vi "MSScript_Act_BlockComment.vi"(8 "error in (no error)":errorcluster, 11 "MSScript in":refnum<class "MSScript.lvclass">) -> (0 "error out":errorcluster, 3 "MSScript out":refnum<class "MSScript.lvclass">)   [LabVIEW 2018, in "MSScript.lvclass"]
uses:
  MSScript.lvclass
  MSScript.lvclass/MSScript.ctl
  MSScript_Error_(6010)CommentLost.vi
  <vilib>/regexp/Match Regular Expression.xnode
panel:
  out "Array":string[](array[string])
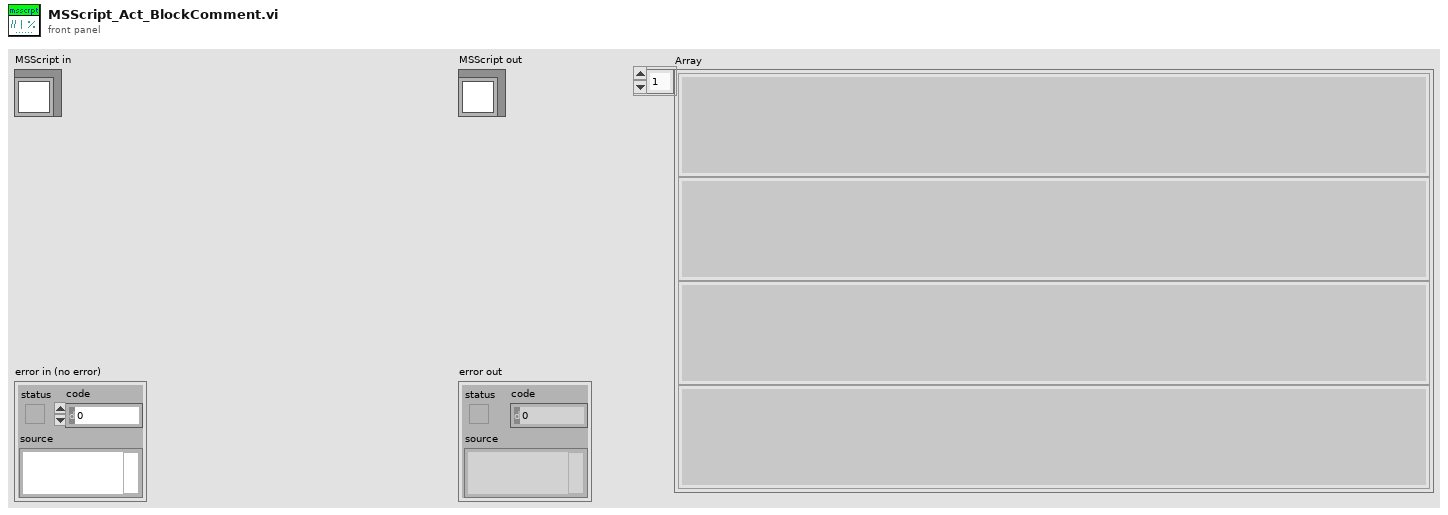
[diagram p1: front panel]
types:
  T1 = cluster{"Colour":u32, "Italic":bool, "Bold":bool}
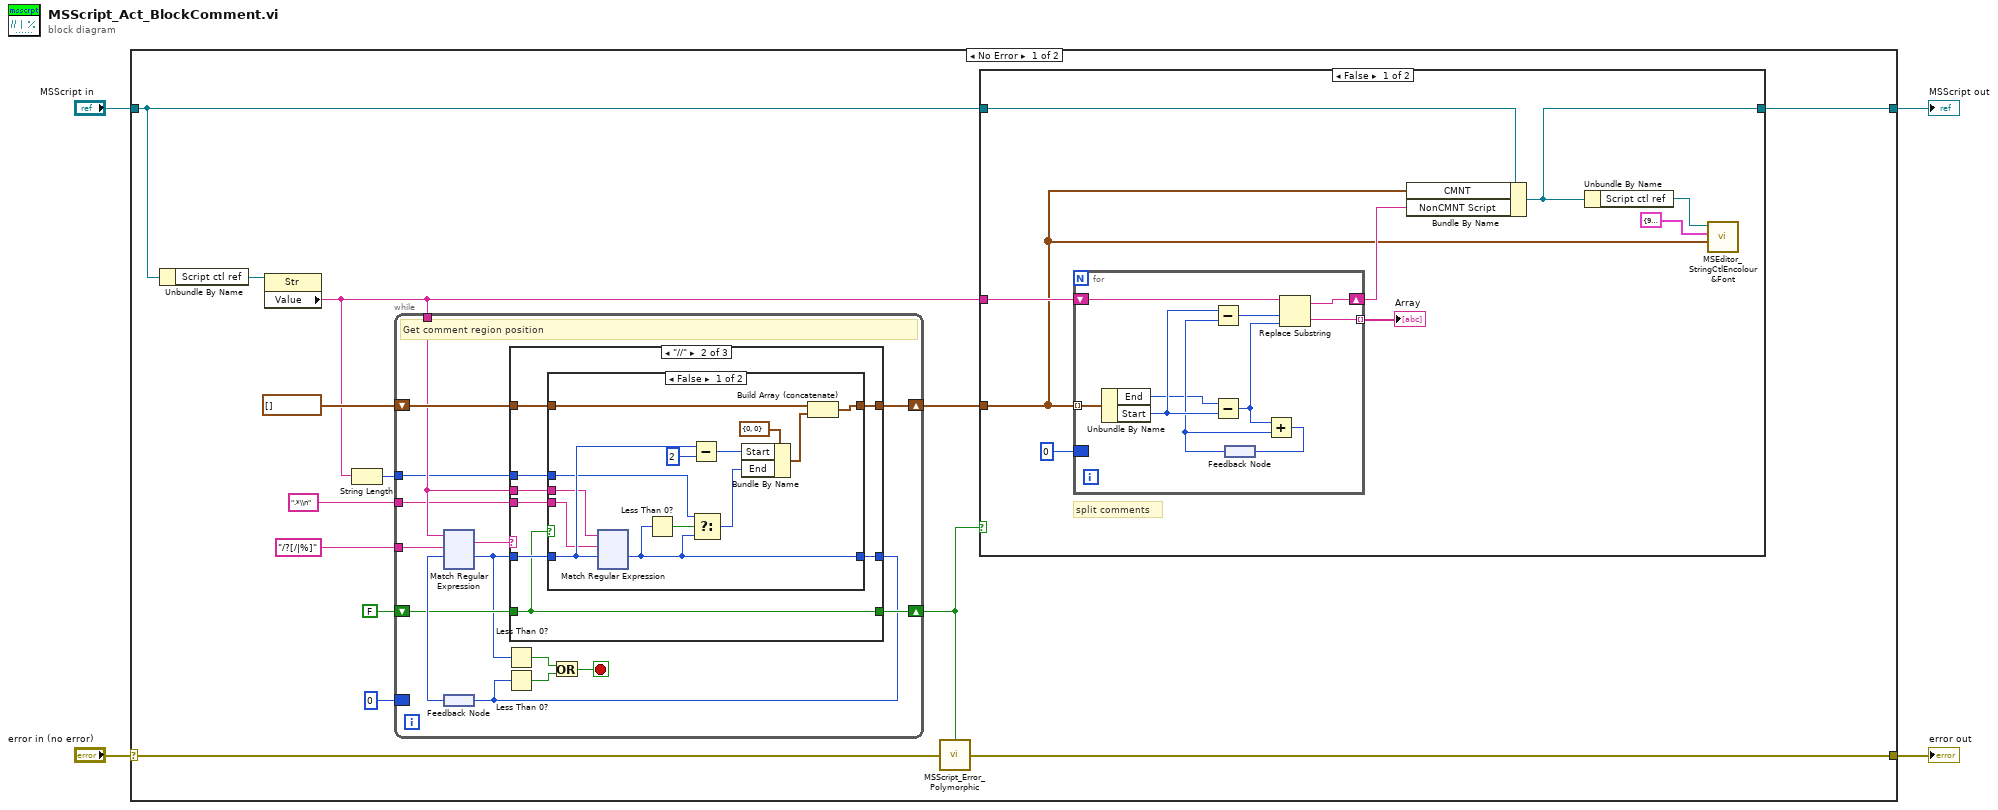
[diagram p0: block diagram]
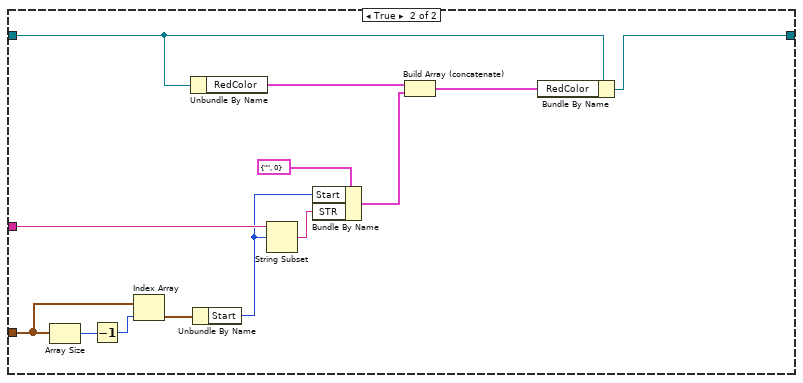
[diagram p2: hidden frame]
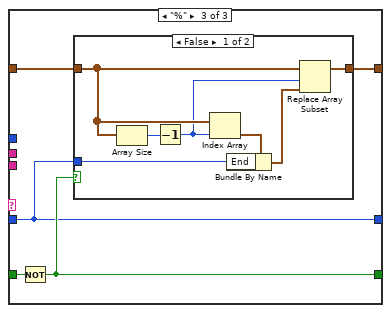
[diagram p5: hidden frame]
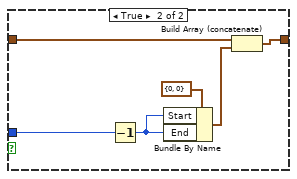
[diagram p6: hidden frame]
diagram:
  n1 = case shown="No Error" "error in (no error)" {
    selector: "error in (no error)" -> [w9 w339]
    tunnel: [w8 w339] -> w3
    tunnel: [w7 w338] -> w1
    tunnel: "MSScript in" -> [w6 w338]
    frame No Error {
      n2 = Unbundle By Name(w6) -> ("Script ctl ref"=w18:refnum<vi>)
      n3 = property class="Str"(reference=w18) -> ("Value"=w11:string)  [unwired: 1 in, 2 out]
      n4 = String Length(string=w11) -> (length=w12:i32)
      n5 = while {
        border: 0 ("offset past match") -> [_]
        tunnel: "/?[/|%]" ("regular expression") -> [w64]
        shift-right: [w61] -> w5
        shift-left: FALSE -> [w62]
        shift-right: [w58] -> w10
        shift-left: cluster{"Start":i32, "End":i32}[] [] ("Comments") -> [w60]
        tunnel: w11 -> [w57]
        tunnel: ".*\\n" ("regular expression") -> [w56]
        tunnel: w12 -> [w55]
        stop <- w51 stop-if-true
        # "Get comment region position"
        n6 = feedback #1() -> (w65:i32)
        n7 = xnode "Match Regular Expression"("input string"=w57, "regular expression"=w64, "offset (0)"=w65) -> ("whole match"=w63:string, "offset past match"=w59:i32)  [unwired: 3 in, 3 out]
        n8 = Less Than 0?(x=w59) -> (x < 0?=w53:bool)
        n9 = case shown="\"//\"" w63 {
          tunnel: w62 -> [w67 w71 w210]
          tunnel: [w67 w71 w209] -> w61
          tunnel: w60 -> [w66 w75 w207]
          tunnel: w57 -> [_ w76 _]
          tunnel: w59 -> [w68 w73 w208]
          tunnel: [w68 w72 w208] -> w54
          tunnel: [w66 w74 w206] -> w58
          tunnel: w56 -> [_ w70 _]
          tunnel: w55 -> [_ w69 _]
          frame "/", Default {
          }
          frame "//" {
            n10 = case shown="False" w71 {
              tunnel: w76 -> [w79 _]
              tunnel: w75 -> [w88 w204]
              tunnel: [w86 w204] -> w74
              tunnel: w73 -> [w85 w205]
              tunnel: [w80 w205] -> w72
              tunnel: w70 -> [w82 _]
              tunnel: w69 -> [w77 _]
              frame False {
                n11 = xnode "Match Regular Expression"("input string"=w79, "regular expression"=w82, "offset (0)"=w85) -> ("offset past match"=w80:i32)  [unwired: 3 in, 4 out]
                n12 = Less Than 0?(x=w80) -> (x < 0?=w81:bool)
                n13 = Subtract(x=w85, y=2) -> (x-y=w83:i32)
                n14 = Select(t=w77, s=w81, f=w80) -> (s? t:f=w78:i32)
                n15 = Bundle By Name(cluster=cluster{"Start":i32, "End":i32} {"Start"=0, "End"=0} ("Location"), "Start"=w83, "End"=w78) -> (w87:cluster{"Start":i32, "End":i32})
                n16 = Build Array (concatenate)(w88, w87) -> (w86:cluster{"Start":i32, "End":i32}[])
              }
              frame True {
              }
            }
          }
          frame "%" {
            n17 = Not(x=w210) -> (.not. x?=w209:bool)
            n18 = case shown="False" w209 {
              tunnel: w208 -> [w215 w221]
              tunnel: w207 -> [w214 w220]
              tunnel: [w211 w219] -> w206
              frame False {
                n19 = Array Size(array=w214) -> (size(s)=w217:i32)
                n20 = Decrement(x=w217) -> (x-1=w212:i32)
                n21 = Index Array(array=w214, index=w212) -> (element=w216:cluster{"Start":i32, "End":i32})
                n22 = Bundle By Name(cluster=w216, "End"=w215) -> (w213:cluster{"Start":i32, "End":i32})
                n23 = Replace Array Subset(array=w214, new element=w213, index=w212) -> (w211:cluster{"Start":i32, "End":i32}[])
              }
              frame True {
                n24 = Decrement(x=w221) -> (x-1=w223:i32)
                n25 = Bundle By Name(cluster=cluster{"Start":i32, "End":i32} {"Start"=0, "End"=0} ("Location"), "Start"=w223, "End"=w223) -> (w218:cluster{"Start":i32, "End":i32})
                n26 = Build Array (concatenate)(w220, w218) -> (w219:cluster{"Start":i32, "End":i32}[])
              }
            }
          }
        }
        n27 = feedback-in #1(w54) -> ()
        n28 = Less Than 0?(x=w54) -> (x < 0?=w52:bool)
        n29 = Or(x=w53, y=w52) -> (x .or. y?=w51:bool)
      }
      n30 = call-poly "MSScript_Error_Polymorphic.vi"("error in (no error)"=w9, "ErrBoolean"=w5) -> ("error out"=w8:errorcluster)
      n31 = case shown="False" w5 {
        tunnel: w11 -> [w24 w42]
        tunnel: w10 -> [w21 w46]
        tunnel: [w20 w47] -> w7
        tunnel: w6 -> [w19 w49]
        frame False {
          # "split comments"
          n32 = for {
            tunnel: w21 -> [w31] mode=indexing
            border: 0 -> [_]
            tunnel: [w34] -> w26 mode=indexing
            shift-right: [w33] -> w25
            shift-left: w24 -> [w32]
            n33 = Unbundle By Name(w31) -> ("End"=w28:i32, "Start"=w30:i32)
            n34 = Subtract(x=w28, y=w30) -> (x-y=w36:i32)
            n35 = feedback #2() -> (w29:i32)
            n36 = Subtract(x=w30, y=w29) -> (x-y=w37:i32)
            n37 = Add(x=w36, y=w29) -> (x+y=w35:i32)
            n38 = feedback-in #2(w35) -> ()
            n39 = Replace Substring(2:w36, 3:w37, 5:w32) -> (0:w34:string, 1:w33:string)  [unwired: 1 in]
          }
          "Array" <- w26
          n40 = Bundle By Name(cluster=w19, "CMNT"=w21, "NonCMNT Script"=w25) -> (w20:refnum<class "MSScript.lvclass">)
          n41 = Unbundle By Name(w20) -> ("Script ctl ref"=w23:refnum<vi>)
          n42 = call "MSEditor_StringCtlEncolour&Font.vi"("SELs"=w21, "TextProperties"=T1 {"Colour"=9868950, "Italic"=TRUE, "Bold"=FALSE}, "String ctl ref"=w23) -> ()  [unwired: 7 in, 2 out]
        }
        frame True {
          n43 = Array Size(array=w46) -> (size(s)=w45:i32)
          n44 = Decrement(x=w45) -> (x-1=w44:i32)
          n45 = Index Array(array=w46, index=w44) -> (element=w43:cluster{"Start":i32, "End":i32})
          n46 = Unbundle By Name(w49) -> ("RedColor"=w50:cluster{"STR":string, "Start":i32}[])
          n47 = Unbundle By Name(w43) -> ("Start"=w39:i32)
          n48 = String Subset(string=w42, offset (0)=w39) -> (substring=w40:string)  [unwired: 1 in]
          n49 = Bundle By Name(cluster=cluster{"STR":string, "Start":i32} {"STR"="", "Start"=0} ("PARAM"), "Start"=w39, "STR"=w40) -> (w38:cluster{"STR":string, "Start":i32})
          n50 = Build Array (concatenate)(w50, w38) -> (w48:cluster{"STR":string, "Start":i32}[])
          n51 = Bundle By Name(cluster=w49, "RedColor"=w48) -> (w47:refnum<class "MSScript.lvclass">)
        }
      }
    }
    frame Error {
    }
  }
  "error out" <- w3
  "MSScript out" <- w1
